vi "Debug Read Peak Current.vi"   [LabVIEW 2010]
uses:
  <instrlib>/Keithley 2400/Keithley 24XX.lvlib
types:
  T1 = enum16{"--Disconnect All--", "Connect PulseGen to CH1", "Connect PulseGen to CH2", "Connect PulseGen to CH3", "Connect PulseGen to CH4", "Connect PulseGen to CH5", "Connect PulseGen to CH6", "Connect PulseGen to CH7", "Connect PulseGen to CH8", "Connect PulseGen to CH9", "Connect PulseGen to CH10", "Connect PulseGen to CH11", "Connect PulseGen to CH12", "Connect PulseGen to CH13", "Connect PulseGen to CH14", "Connect PulseGen to CH15", "Connect PulseGen to CH16", "Connect PulseGen to CH17", "Connect PulseGen to CH18", "Connect PulseGen to CH19", "Connect PulseGen to CH20", "Connect PulseGen to CH21", "Connect PulseGen to CH22", "Connect PulseGen to CH23", "Connect PulseGen to CH24", "Connect PulseGen to CH25", "Set MAG_SW", "Set Dynamic Load", "Set Expansion Trigger", "Trigger Positive Pulse", "Trigger Negative Pulse", "Set MSP Magic Pin", "Set BAT_EN", "Connect MSP_ACLK to CTR", "Connect MSP_MCLK to CTR", "Connect MSP_DIG_TST_OUT to CTR", "Connect STIM_SCK to CTR", "Connect STIM_CLK to CTR", "Connect SMU2 to Magnet", "Magnet Enable", "Cap Short", "Connect Positive Pulse to Pulse Bus", "Connect Negative Pulse to Pulse Bus", "Connect JTAG", "Connect JTAG DVDD Power", "RF Attach", "Connect SMU3 to VBAT", "Connect SMU3 Soft Start", "Connect ARB to Charge Coil", "Connect ARB to Matrix", "Connect CTR to Matrix", "DMM_I Short", "DMM_I 1000 Ohm", "DMM_I 100 Ohm", "DMM_I 10 Ohm", "Connect CH25 to DUT GND"}
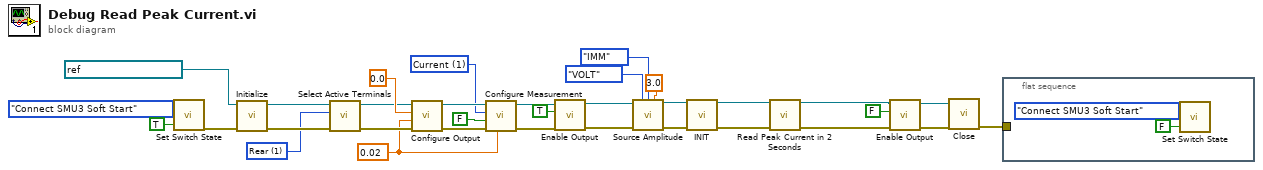
[diagram p0: block diagram]
diagram:
  w23 = u16 1 items=["Volts", "Current", "Resistance"] ("Function (0: Volts)")
  w26 = u16 1 items=["Front", "Rear"] ("Active Terminals (0: Front)")
  w19 = 0.02 ("Compliance  Level (0.1)")
  n1 = call "Set Switch State.vi"("Action"=T1."Connect SMU3 Soft Start", "State"=TRUE) -> ("error out"=w16:errorcluster)  [unwired: 13 in]
  n2 = call <instrlib>:"Initialize.vi"("error in (no error)"=w16, "VISA resource name"=refnum<visa-resource-name> "GPIB0::6::INSTR") -> ("error out"=w28:errorcluster, "VISA resource name out"=w30:refnum<visa-resource-name>)  [unwired: 8 in]
  n3 = call <instrlib>:"Select Active Terminals.vi"("error in (no error)"=w28, "Active Terminals (0: Front)"=w26, "VISA resource name"=w30) -> ("error out"=w27:errorcluster, "VISA resource name out"=w29:refnum<visa-resource-name>)  [unwired: 7 in]
  n4 = call <instrlib>:"Configure Output.vi"("error in (no error)"=w27, "Compliance  Level (0.1)"=w19, "Output Level (0)"=0.0, "VISA resource name"=w29) -> ("error out"=w24:errorcluster, "VISA resource name out"=w25:refnum<visa-resource-name>)  [unwired: 6 in]
  n5 = call <instrlib>:"Configure Measurement.vi"("Manual Range (1.0)"=w19, "error in (no error)"=w24, "Enable Auto Range (T:Enable)"=FALSE, "Function (0: Volts)"=w23, "VISA resource name"=w25) -> ("error out"=w20:errorcluster, "VISA resource name out"=w21:refnum<visa-resource-name>)  [unwired: 5 in]
  n6 = call <instrlib>:"Enable Output.vi"("error in (no error)"=w20, "Enable Output (T: Enable)"=TRUE, "VISA resource name"=w21) -> ("error out"=w8:errorcluster, "VISA resource name out"=w9:refnum<visa-resource-name>)  [unwired: 7 in]
  n7 = call "Source Amplitude.vi"("VISA resource name"=w9, "Source Function"=enum16{"CURR", "VOLT"}."VOLT", "Mode"=enum16{"IMM", "TRIGGERED"}."IMM", "Source Level"=3.0, "error in (no error)"=w8) -> ("VISA resource name out"=w15:refnum<visa-resource-name>, "error out"=w14:errorcluster)  [unwired: 9 in]
  n8 = call "INIT.vi"("VISA resource name"=w15, "error in (no error)"=w14) -> ("VISA resource name out"=w5:refnum<visa-resource-name>, "error out"=w4:errorcluster)  [unwired: 12 in]
  n9 = call "Read Peak Current in 2 Seconds.vi"("VISA resource name"=w5, "error in (no error)"=w4) -> ("VISA resource name out"=w3:refnum<visa-resource-name>, "error out"=w2:errorcluster)  [unwired: 11 in, 1 out]
  n10 = call <instrlib>:"Enable Output.vi"("error in (no error)"=w2, "Enable Output (T: Enable)"=FALSE, "VISA resource name"=w3) -> ("error out"=w10:errorcluster, "VISA resource name out"=w11:refnum<visa-resource-name>)  [unwired: 7 in]
  n11 = call <instrlib>:"Close.vi"("error in (no error)"=w10, "VISA resource name"=w11) -> ("error out"=w1:errorcluster)  [unwired: 9 in]
  n12 = flat-sequence {
    tunnel: w1 -> [_]
    frame #0 {
      n13 = call "Set Switch State.vi"("Action"=T1."Connect SMU3 Soft Start", "State"=FALSE) -> ()  [unwired: 13 in, 1 out]
    }
  }
